vi "tearDown.vi"(8 "error in (no error)":errorcluster, 11 "reference in":refnum<class "Logging Loopback.lvclass">) -> (0 "error out":errorcluster, 3 "reference out":refnum<class "Logging Loopback.lvclass">)   [LabVIEW 2020, in "Logging Loopback.lvclass"]
doc: "tearDown runs after the test method has completed. Use this method to clean up any operations or references that were opened by setUp or the test method. Unit tests should be independent of other unit tests so this VI should ensure that the next test can run in a 'clean' test environment."
uses:
  Logging Loopback.lvclass
  Logging Loopback.lvclass/Logging Loopback.ctl
  <vilib>/WebDAVClient/NI_WebDAV.lvlib
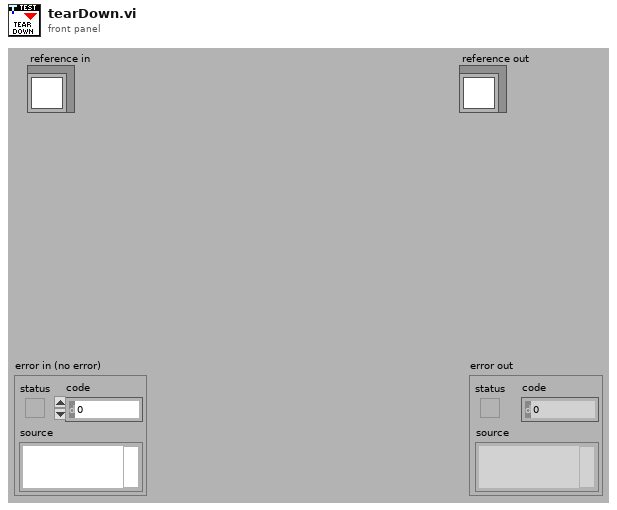
[diagram p1: front panel]
types:
  T1 = typedef "NI_WebDAV.lvlib/SessionHandle.ctl" = refnum<k1>
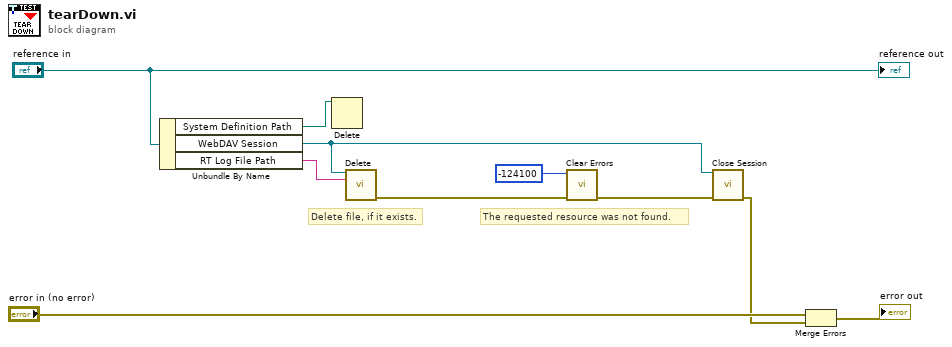
[diagram p0: block diagram]
diagram:
  # "Delete file, if it exists."
  # "The requested resource was not found."
  n1 = Unbundle By Name("reference in") -> ("System Definition Path"=w1:path, "WebDAV Session"=w3:T1, "RT Log File Path"=w5:string)
  n2 = Delete(path (use dialog)=w1) -> ()  [unwired: 4 in, 3 out]
  n3 = call <vilib>:"Delete.vi"("session handle"=w3, "relative uri"=w5) -> ("error out"=w7:errorcluster)  [unwired: 12 in, 1 out]
  n4 = call <vilib>:"Clear Errors.vi"("error in (no error)"=w7, "specific error code to clear (0: all)"=-124100) -> ("error out"=w4:errorcluster)  [unwired: 4 in, 1 out]
  n5 = call <vilib>:"Close Session.vi"("session handle"=w3, "error in (no error)"=w4) -> ("error out"=w2:errorcluster)  [unwired: 13 in]
  n6 = Merge Errors("error in (no error)", w2) -> (→"error out":errorcluster)
  "reference out" <- "reference in"
